vi "Load ALL Ports.vi"(0 "path":path) -> (1 "VALID":bool, 2 "VM Cluster":T3, 3 "VP Cluster":T2, 4 "CA Cluster":T1)   [LabVIEW 2010]
panel:
  out "VM Output Names":string[](array[string])
  out "VM Input Names":string[](array[string])
  out "VM Input Numbers":i32[](array[numeric])
  out "VP Input Names":string[](array[string])
  out "VP Output Names":string[](array[string])
  out "CA Output Numbers":i32[](array[numeric])
  out "CA Input Numbers":i32[](array[numeric])
  out "CA Output Names":string[](array[string])
  out "CA Input Names":string[](array[string])
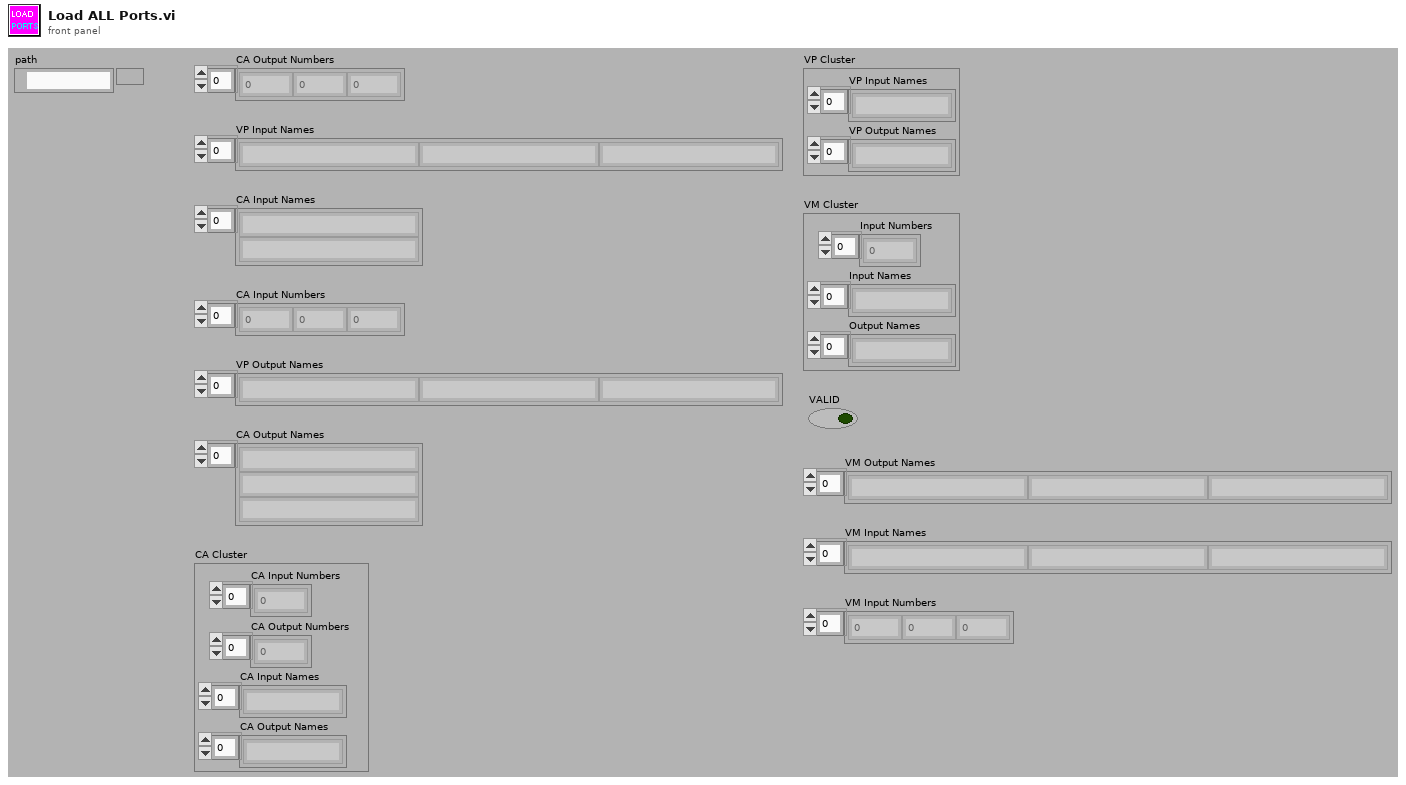
[diagram p1: front panel]
types:
  T1 = cluster{"CA Input Numbers":i32[], "CA Output Numbers ":i32[], "CA Input Names":string[], "CA Output Names ":string[]}
  T2 = cluster{"VP Input Names":string[], "VP Output Names ":string[]}
  T3 = cluster{"Input Numbers":i32[], "Input Names":string[], "Output Names ":string[]}
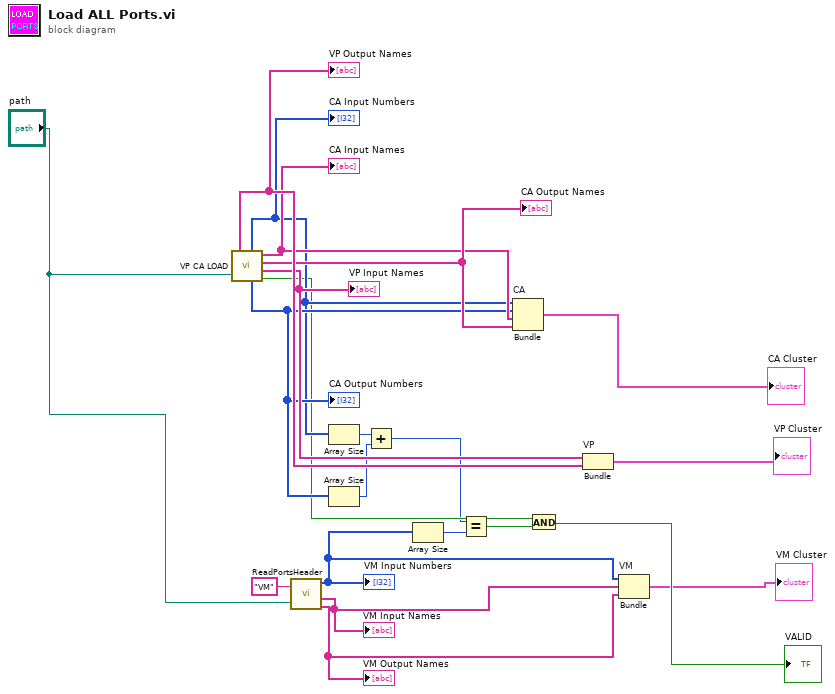
[diagram p0: block diagram]
diagram:
  n1 = call "VP CA LOAD.vi"("path"="path") -> ("VP Output Names"=w15:string[], "CA Output Numbers"=w10:i32[], "CA Input Numbers"=w9:i32[], "VALID"=w8:bool, "VP Input Names"=w14:string[], "CA Output Names"=w12:string[], "CA Input Names"=w11:string[])
  "CA Input Names" <- w11
  "CA Output Names" <- w12
  "CA Input Numbers" <- w9
  "CA Output Numbers" <- w10
  "VP Output Names" <- w15
  "VP Input Names" <- w14
  n2 = call "ReadPortsHeader.vi"("base path"="path", "FileName"="VM" ("name or relative path")) -> ("Output Names"=w19:string[], "Input Names"=w18:string[], "Input Numbers"=w17:i32[])  [unwired: 1 out]
  "VM Input Numbers" <- w17
  "VM Input Names" <- w18
  "VM Output Names" <- w19
  n3 = Array Size(array=w9) -> (size(s)=w3:i32)
  n4 = Array Size(array=w10) -> (size(s)=w4:i32)
  n5 = Add(x=w3, y=w4) -> (x+y=w6:i32)
  n6 = Array Size(array=w17) -> (size(s)=w5:i32)
  n7 = Equal?(x=w6, y=w5) -> (x = y?=w7:bool)
  n8 = Bundle "CA"("CA Input Numbers"=w9, "CA Output Numbers"=w10, "CA Input Names"=w11, "CA Output Names"=w12) -> (→"CA Cluster":T1)  [unwired: 1 in]
  n9 = And(x=w8, y=w7) -> (x .and. y?=→"VALID":bool)
  n10 = Bundle "VP"("VP Input Names"=w14, "VP Output Names"=w15) -> (→"VP Cluster":T2)  [unwired: 1 in]
  n11 = Bundle "VM"("Input Numbers"=w17, "Input Names"=w18, "Output Names"=w19) -> (→"VM Cluster":T3)  [unwired: 1 in]
